vi "parseDataU8.vi"(8 "error in (no error)":errorcluster, 11 "FrameParser in":refnum<class "FrameParser.lvclass">) -> (0 "error out":errorcluster, 2 "Data":u8, 3 "FrameParser out":refnum<class "FrameParser.lvclass">)   [LabVIEW 2015, in "FrameParser.lvclass"]
uses:
  FrameParser.lvclass
  FrameParser.lvclass/FrameParser.ctl
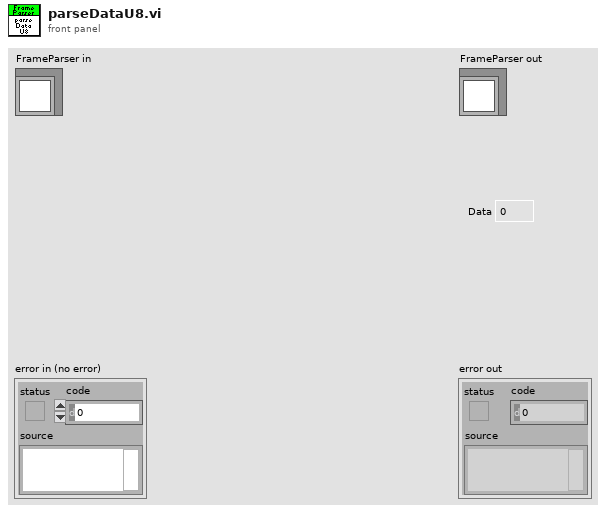
[diagram p1: front panel]
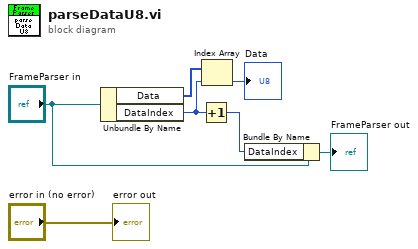
[diagram p0: block diagram]
diagram:
  n1 = Unbundle By Name("FrameParser in") -> ("Data"=w7:u8[], "DataIndex"=w3:i32)
  n2 = Increment(x=w3) -> (x+1=w2:i32)
  n3 = Index Array(array=w7, index=w3) -> (element=→"Data":u8)
  n4 = Bundle By Name(cluster="FrameParser in", "DataIndex"=w2) -> (→"FrameParser out":refnum<class "FrameParser.lvclass">)
  "error out" <- "error in (no error)"
